vi "Get Last Row, Column.vi"(8 "error in (no error)":errorcluster, 10 "Sheet Reference":refnum<k24>) -> (0 "error out":errorcluster, 2 "Sheet Reference out":refnum<k24>, 4 "Last Column":i32, 5 "Last Row":i32)   [LabVIEW 2013]
doc: "Returns the last row and column. These numbers are zero-based."
uses:
  C:/PhaeronGit/LVNPOI/Resources/NPOI 2.1.1 dotnet2/NPOI.dll
  Resources/NPOI 2.1.1 dotnet2/NPOI.dll
panel:
  # "These are zero-based."
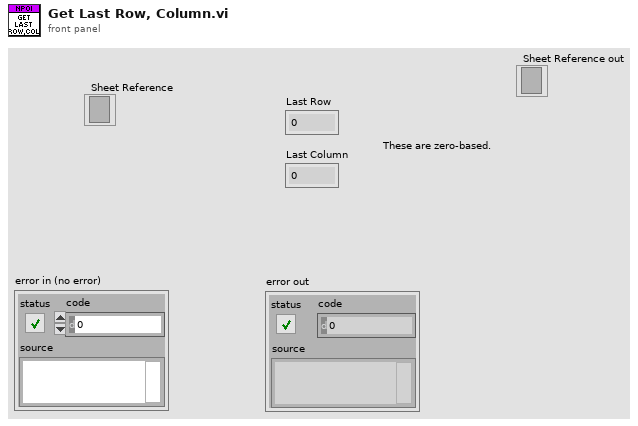
[diagram p1: front panel]
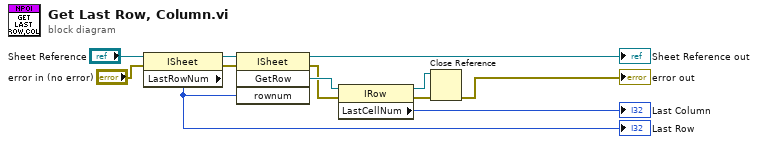
[diagram p0: block diagram]
diagram:
  n1 = property class="ISheet"(reference="Sheet Reference", error in="error in (no error)") -> (reference out=w9:refnum<k24>, error out=w10:errorcluster, "LastRowNum"=w1:i32)
  "Last Row" <- w1
  n2 = invoke class="ISheet" method="GetRow"(reference=w9, error in=w10, "rownum"=w1) -> (reference out=→"Sheet Reference out":refnum<k24>, error out=w7:errorcluster, "GetRow"=w8:refnum<k24>)  [unwired: 1 in, 1 out]
  n3 = property class="IRow"(reference=w8, error in=w7) -> (reference out=w3:refnum<k24>, error out=w4:errorcluster, "LastCellNum"=→"Last Column":i16)
  n4 = Close Reference(reference=w3, error in (no error)=w4) -> (error out=→"error out":errorcluster)
